vi "Add point to array for XY graph.vi"(0 "X-axis":dbl, 1 "Write?(T)":bool=TRUE, 2 "Input A":dbl, 3 "Input B":dbl, 4 "Reset?(F)":bool) -> (6 "Array":cluster{"Array":dbl[], "Array":dbl[]}[](array[cluster]))   [LabVIEW 2024]
panel:
  out "size":i32
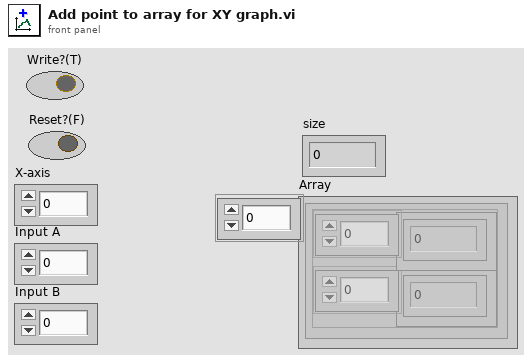
[diagram p1: front panel]
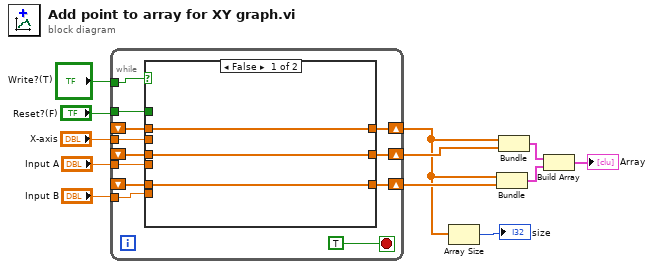
[diagram p0: block diagram]
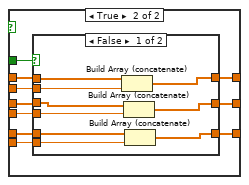
[diagram p2: hidden frame]
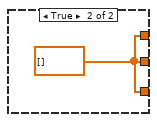
[diagram p3: hidden frame]
diagram:
  n1 = while {
    tunnel: "X-axis" -> [w20]
    tunnel: "Input A" -> [w19]
    tunnel: "Input B" -> [w16]
    shift-right: [w23] -> w3
    shift-left: _ -> [w21]
    shift-right: [w22] -> w8
    shift-left: _ -> [w18]
    shift-right: [w24] -> w9
    shift-left: _ -> [w17]
    tunnel: "Reset?(F)" -> [w14]
    tunnel: "Write?(T)" -> [w13]
    stop <- TRUE stop-if-true
    n2 = case shown="False" w13 {
      tunnel: [w25 w37] -> w24
      tunnel: [w27 w36] -> w23
      tunnel: [w26 w35] -> w22
      tunnel: w21 -> [w27 w34]
      tunnel: w20 -> [_ w33]
      tunnel: w19 -> [_ w32]
      tunnel: w18 -> [w26 w31]
      tunnel: w17 -> [w25 w30]
      tunnel: w16 -> [_ w29]
      tunnel: w14 -> [_ w28]
      frame False {
      }
      frame True {
        n3 = case shown="False" w28 {
          tunnel: [w46 w47] -> w37
          tunnel: [w45 w47] -> w36
          tunnel: [w44 w47] -> w35
          tunnel: w34 -> [w43 _]
          tunnel: w33 -> [w42 _]
          tunnel: w32 -> [w41 _]
          tunnel: w31 -> [w40 _]
          tunnel: w30 -> [w39 _]
          tunnel: w29 -> [w38 _]
          frame False {
            n4 = Build Array (concatenate)(w43, w42) -> (w45:dbl[])
            n5 = Build Array (concatenate)(w40, w41) -> (w44:dbl[])
            n6 = Build Array (concatenate)(w39, w38) -> (w46:dbl[])
          }
          frame True {
            w47 = dbl[] []
          }
        }
      }
    }
  }
  n7 = Array Size(array=w3) -> (size(s)=→"size":i32)
  n8 = Bundle(w3, w9) -> (w10:cluster{dbl[], dbl[]})  [unwired: 1 in]
  n9 = Bundle(w3, w8) -> (w11:cluster{dbl[], dbl[]})  [unwired: 1 in]
  n10 = Build Array(w11, w10) -> (→"Array":cluster{dbl[], dbl[]}[])
